vi "AudioTest.Run SoundCheck Sequence.vi"(7 "Config":T1={"SeqDir"=path "C:/MTE/Audio Test/Config/SoundCheck/Sequences", "SoundCheckApp"=path "C:/SoundCheck 16.0-x64/SoundCheck 16.0 (x64).exe", "IP"="localhost", "Port"=4444, "Process Name"="SoundCheck 16.0 (x64)", "DataDir"=path "C:/MTE/Audio Test/Data/SoundCheck", "Window"=enum."Normal"}, 8 "error in":errorcluster, 9 "UUT Dir":path, 10 "Timeout(s)":dbl=60.0, 11 "Sequence":string="UTAH_EV2_SEQUENCE_20180820_DUMMY2.sqc") -> (0 "error out":errorcluster, 1 "App Launch Dur(s)":dbl, 2 "Duration":dbl, 3 "Ran to completion":bool)   [LabVIEW 2018]
uses:
  TypeDefs/SoundCheck Config.ctl
  Common/Utils/Errors/Error.Error Code List.ctl
  <vilib>/KATE/Files/File Utils.lvlib
  <vilib>/KATE/Time/Time Utils.lvlib
panel:
  out "Status":string
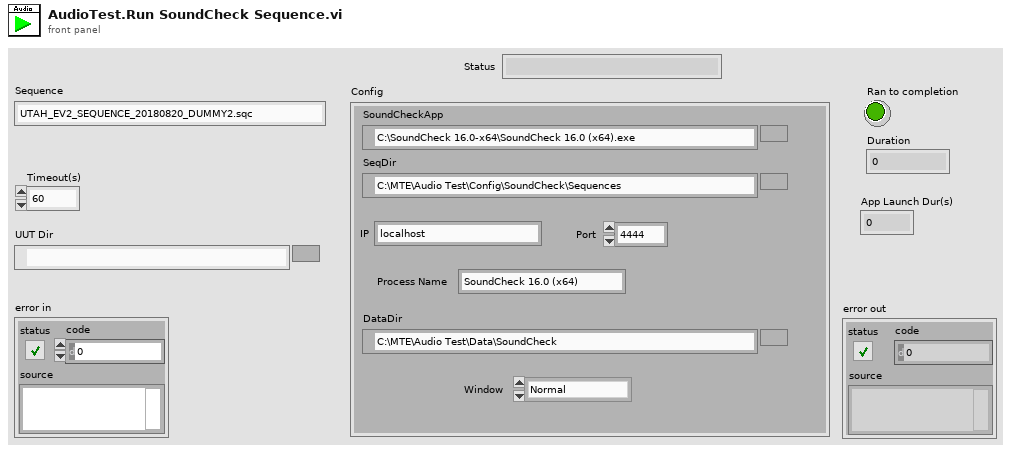
[diagram p1: front panel]
types:
  T1 = typedef "SoundCheck Config.ctl" = cluster{"SeqDir":path, "SoundCheckApp":path, "IP":string, "Port":u16, "Process Name":string, "DataDir":path, "Window":enum16{"Normal", "Minimized", "Hidden"}}
  T2 = typedef "Error.Error Code List.ctl" = i32
  T3 = cluster{"Config":T1, "Sequence":string, "Timeout(s)":dbl, "UUT Dir":path}
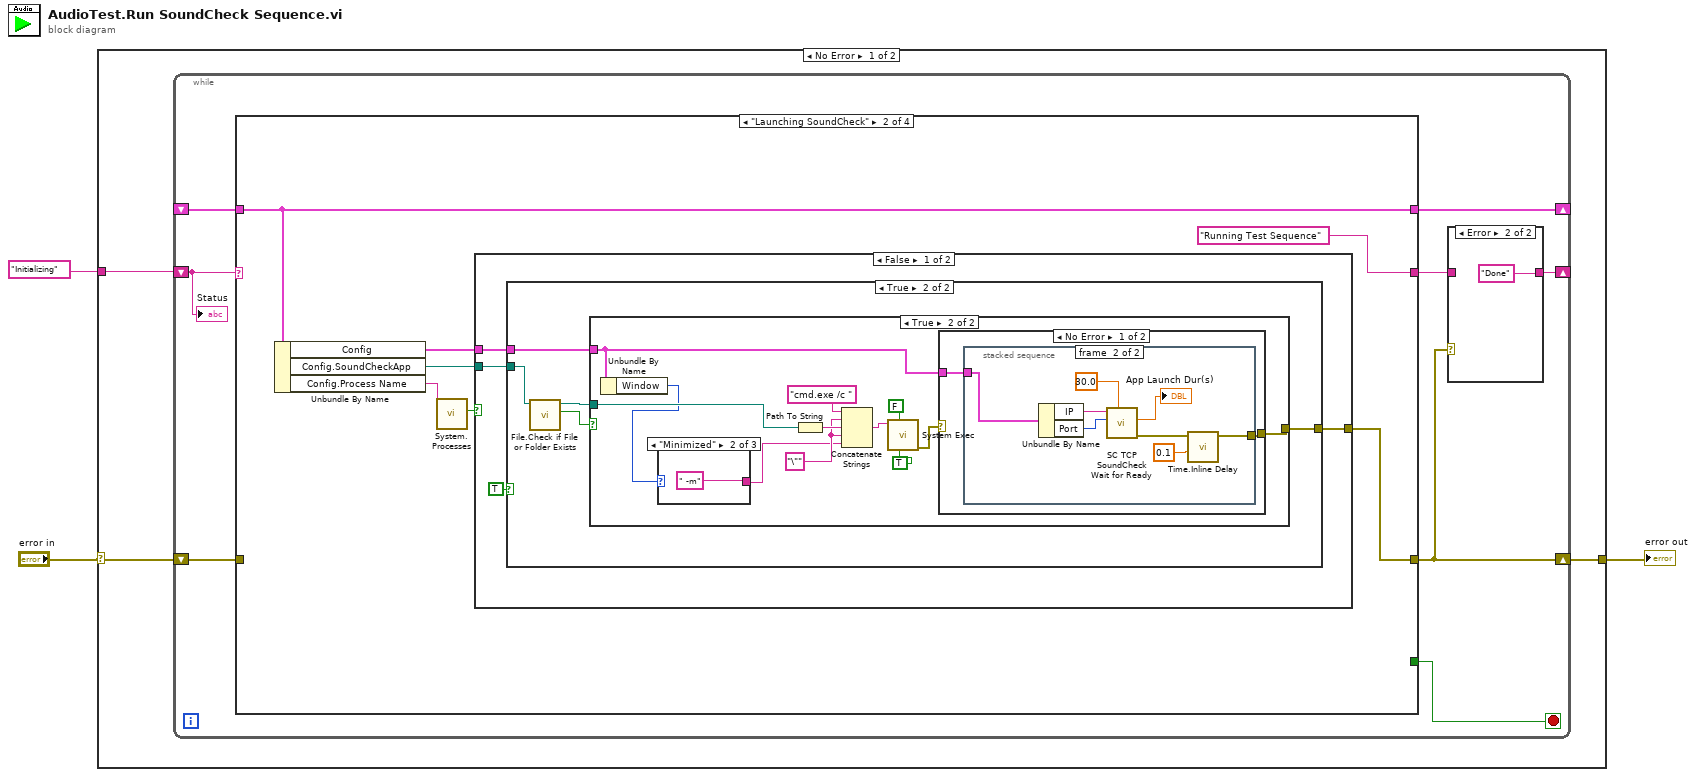
[diagram p0: block diagram]
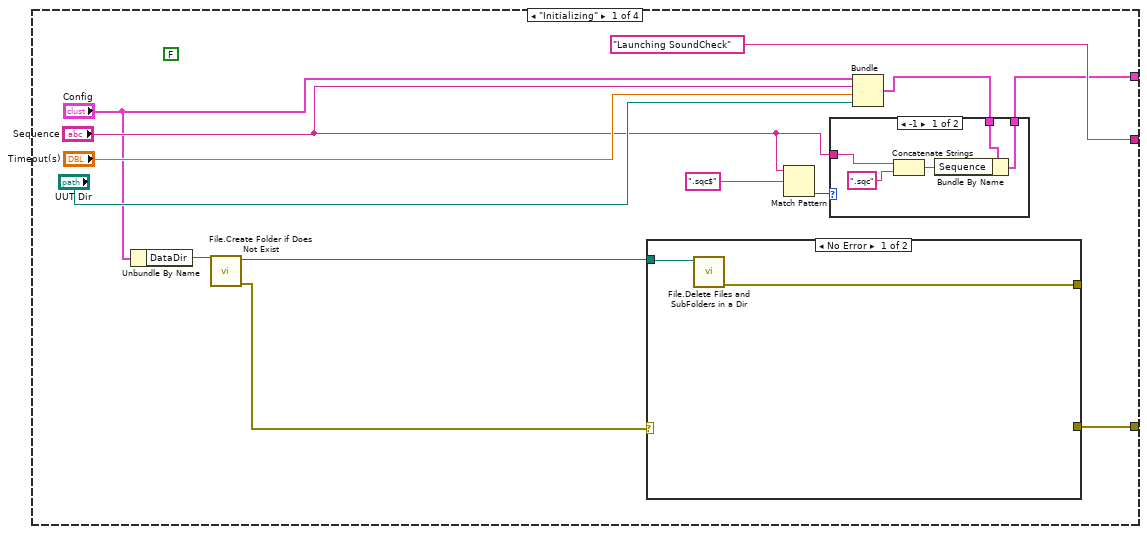
[diagram p3: hidden frame]
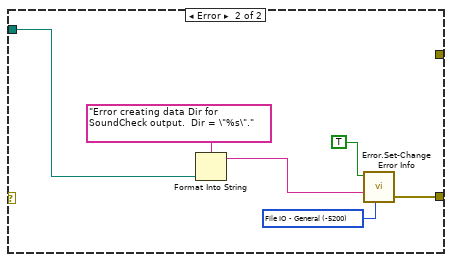
[diagram p5: hidden frame]
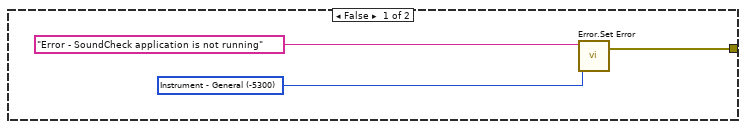
[diagram p6: hidden frame]
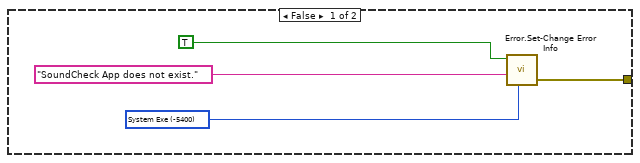
[diagram p7: hidden frame]
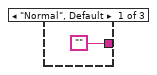
[diagram p8: hidden frame]
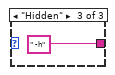
[diagram p9: hidden frame]
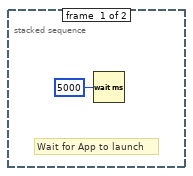
[diagram p10: hidden frame]
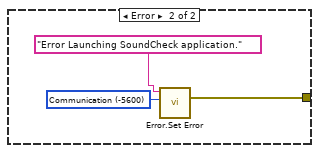
[diagram p11: hidden frame]
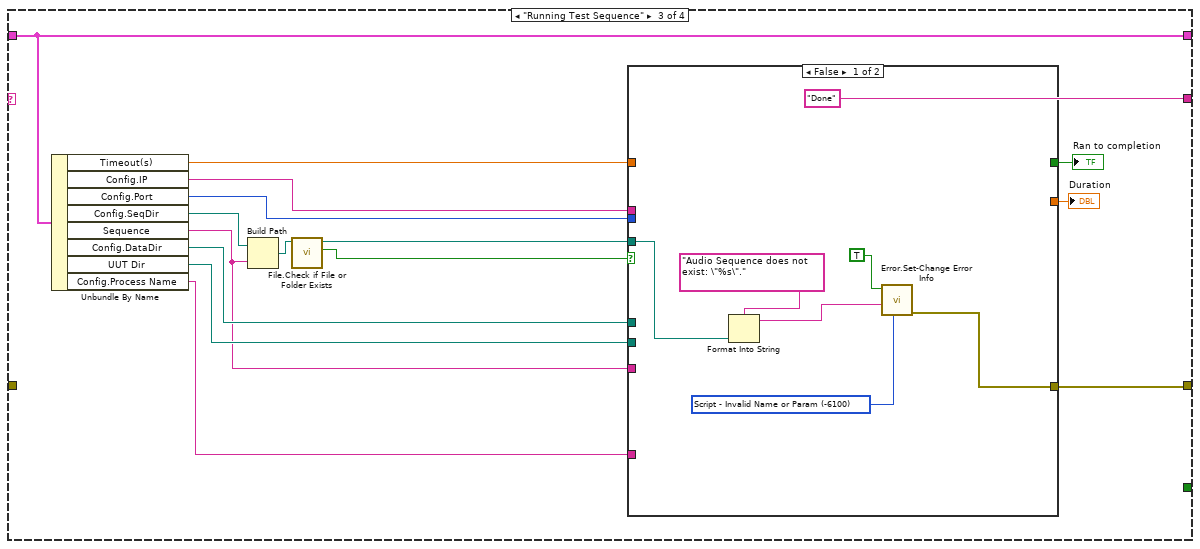
[diagram p13: hidden frame]
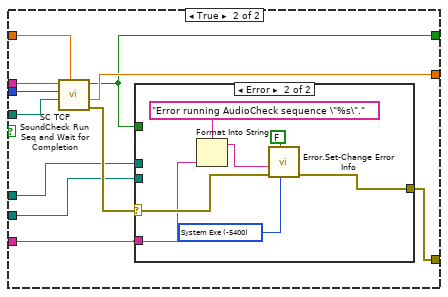
[diagram p14: hidden frame]
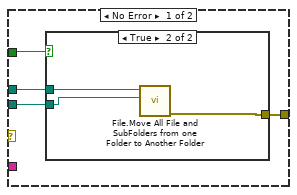
[diagram p15: hidden frame]
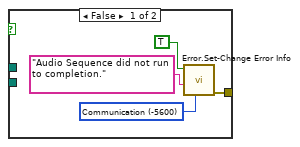
[diagram p16: hidden frame]
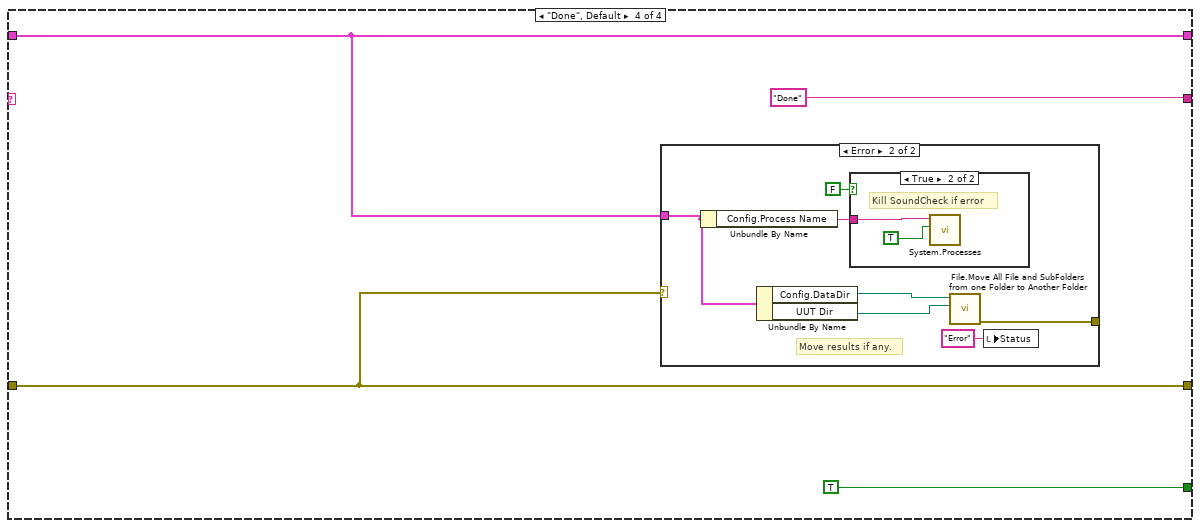
[diagram p17: hidden frame]
diagram:
  n1 = case shown="No Error" "error in" {
    selector: "error in" -> [w5 w160]
    tunnel: [w6 w160] -> w3
    tunnel: "Initializing" -> [w4 _]
    frame No Error {
      n2 = while {
        shift-right: [w14] -> _
        shift-left: _ -> [w13]
        shift-right: [w10] -> w6
        shift-left: w5 -> [w12]
        shift-right: [w8] -> _
        shift-left: w4 -> [w7]
        stop <- w11 stop-if-true
        n3 = case shown="\"Launching SoundCheck\"" w7 {
          tunnel: [w19 w48 w110 w148] -> w14
          tunnel: w13 -> [_ w48 w110 w148]
          tunnel: ["Launching SoundCheck" "Running Test Sequence" "Done" "Done"] -> w9
          tunnel: w12 -> [_ _ _ w147]
          tunnel: [w24 w49 w102 w147] -> w10
          tunnel: [_ _ _ TRUE] -> w11
          frame "Initializing" {
            (unwired) FALSE ("Done")
            n4 = Unbundle By Name("Config") -> ("DataDir"=w26:path)
            n5 = call <vilib>:"File.Create Folder if Does Not Exist.vi"("Path"=w26) -> ("error out"=w25:errorcluster, "Dup Path"=w18:path)  [unwired: 8 in, 1 out]
            n6 = case shown="No Error" w25 {
              tunnel: [_ w41] -> w24
              tunnel: w18 -> [w37 w39]
              tunnel: [w36 _] -> _
              frame No Error {
                n7 = call <vilib>:"File.Delete Files and SubFolders in a Dir.vi"("Dir"=w37) -> ("error out"=w36:errorcluster)  [unwired: 9 in, 1 out]
              }
              frame Error {
                w43 = T2 -5200 items=["No Error"=0, "Abort"=-2, "Misc"=-5000, "Fixture Error"=-5100, "File IO - General"=-5200, "FIle IO - Config Error"=-5201, "Instrument - General"=-5300, "Instrument - Serial Com"=-5301, "Instrument - Camera"=-5302, "Instrument - PS"=-5303, "Instrument - Oscilloscope"=-5304, "Instrument - Function Gen"=-5305, "Instrument - Load"=-5306, "Instrument - Meter"=-5307, "Instrument - Power Control"=-5308, "Instrument - Motion"=-5309, "Instrument - RF"=-5310, "System Exe"=-5400, "Image Processing"=-5500, "Communication"=-5600, "Script - Syntax Error"=-6000, "Script - Invalid Name or Param"=-6100, "Script - Timeout"=-6200, "Invalid Data"=-6300, "FW Update Error"=-6500] ("Std Code")
                n8 = Format Into String(format string="Error creating data Dir for SoundCheck output.  Dir = \"%s\"." ("Description"), w39) -> (resulting string=w38:string)  [unwired: 2 in, 1 out]
                n9 = call "Error.Set-Change Error Info.vi"("Std Code"=w43, "Description"=w38, "Set Error"=TRUE) -> ("error out"=w41:errorcluster)  [unwired: 8 in]
              }
            }
            n10 = Match Pattern(string="Sequence", regular expression=".sqc$") -> (offset past match=w22:i32)  [unwired: 1 in, 3 out]
            n11 = Bundle("Config"="Config", "Sequence"="Sequence", "Timeout(s)"="Timeout(s)", "UUT Dir"="UUT Dir") -> (w20:T3)  [unwired: 1 in]
            n12 = case shown="-1" w22 {
              tunnel: "Sequence" -> [w31 _]
              tunnel: w20 -> [w34 w35]
              tunnel: [w33 w35] -> w19
              frame -1 {
                n13 = Concatenate Strings(w31, ".sqc") -> (w32:string)
                n14 = Bundle By Name(cluster=w34, "Sequence"=w32) -> (w33:T3)
              }
              frame 0, Default {
              }
            }
          }
          frame "Launching SoundCheck" {
            n15 = Unbundle By Name(w48) -> ("Config"=w44:T1, "Config.SoundCheckApp"=w46:path, "Config.Process Name"=w47:string)
            n16 = call "System.Processes.vi"("Process Name"=w47) -> ("Is Running"=w45:bool)  [unwired: 8 in, 2 out]
            n17 = case shown="False" w45 {
              tunnel: [w54 _] -> w49
              tunnel: w46 -> [w53 _]
              tunnel: w44 -> [w52 _]
              frame False {
                n18 = case shown="True" TRUE {
                  tunnel: [w55 w62] -> w54
                  tunnel: w53 -> [_ w61]
                  tunnel: w52 -> [_ w58]
                  frame False {
                    w56 = T2 -5300 items=["No Error"=0, "Abort"=-2, "Misc"=-5000, "Fixture Error"=-5100, "File IO - General"=-5200, "FIle IO - Config Error"=-5201, "Instrument - General"=-5300, "Instrument - Serial Com"=-5301, "Instrument - Camera"=-5302, "Instrument - PS"=-5303, "Instrument - Oscilloscope"=-5304, "Instrument - Function Gen"=-5305, "Instrument - Load"=-5306, "Instrument - Meter"=-5307, "Instrument - Power Control"=-5308, "Instrument - Motion"=-5309, "Instrument - RF"=-5310, "System Exe"=-5400, "Image Processing"=-5500, "Communication"=-5600, "Script - Syntax Error"=-6000, "Script - Invalid Name or Param"=-6100, "Script - Timeout"=-6200, "Invalid Data"=-6300, "FW Update Error"=-6500] ("Std Code")
                    n19 = call "Error.Set Error.vi"("Code"=w56, "Desc"="Error - SoundCheck application is not running") -> ("error out"=w55:errorcluster)  [unwired: 5 in]
                  }
                  frame True {
                    n20 = call <vilib>:"File.Check if File or Folder Exists.vi"("Path"=w61) -> ("Exists"=w59:bool, "Dup Path"=w60:path)  [unwired: 6 in, 3 out]
                    n21 = case shown="True" w59 {
                      tunnel: [w66 w78] -> w62
                      tunnel: w60 -> [_ w70]
                      tunnel: w58 -> [_ w77]
                      frame False {
                        w63 = T2 -5400 items=["No Error"=0, "Abort"=-2, "Misc"=-5000, "Fixture Error"=-5100, "File IO - General"=-5200, "FIle IO - Config Error"=-5201, "Instrument - General"=-5300, "Instrument - Serial Com"=-5301, "Instrument - Camera"=-5302, "Instrument - PS"=-5303, "Instrument - Oscilloscope"=-5304, "Instrument - Function Gen"=-5305, "Instrument - Load"=-5306, "Instrument - Meter"=-5307, "Instrument - Power Control"=-5308, "Instrument - Motion"=-5309, "Instrument - RF"=-5310, "System Exe"=-5400, "Image Processing"=-5500, "Communication"=-5600, "Script - Syntax Error"=-6000, "Script - Invalid Name or Param"=-6100, "Script - Timeout"=-6200, "Invalid Data"=-6300, "FW Update Error"=-6500] ("Std Code")
                        n22 = call "Error.Set-Change Error Info.vi"("Std Code"=w63, "Description"="SoundCheck App does not exist.", "Set Error"=TRUE) -> ("error out"=w66:errorcluster)  [unwired: 8 in]
                      }
                      frame True {
                        w71 = "\"" ("string")
                        n23 = Unbundle By Name(w77) -> ("Window"=w68:enum16{"Normal", "Minimized", "Hidden"})
                        n24 = case shown="\"Minimized\"" w68 {
                          tunnel: ["" " -m" " -h"] -> w69
                          frame "Normal", Default {
                          }
                          frame "Minimized" {
                          }
                          frame "Hidden" {
                          }
                        }
                        n25 = Path To String(path=w70) -> (string=w72:string)
                        n26 = Concatenate Strings("cmd.exe /c ", w71, w72, w71, w69) -> (w76:string)
                        n27 = call <vilib>:"System Exec.vi"("run minimized? (F)"=TRUE, "wait until completion? (T)"=FALSE, "command line"=w76) -> ("error out"=w67:errorcluster)  [unwired: 5 in, 3 out]
                        n28 = case shown="No Error" w67 {
                          tunnel: [w82 w93] -> w78
                          tunnel: w77 -> [w83 _]
                          frame No Error {
                            n29 = stacked-sequence {
                              tunnel: w83 -> [_ w92]
                              tunnel: [_ w87] -> w82
                              frame #0 {
                                # "Wait for App to launch"
                                n30 = Wait (ms)(milliseconds to wait=u32 5000) -> ()  [unwired: 1 out]
                              }
                              frame #1 {
                                n31 = Unbundle By Name(w92) -> ("IP"=w91:string, "Port"=w90:u16)
                                n32 = call "SC TCP SoundCheck Wait for Ready.vi"("TimeOut(s)"=30.0, "port (4444)"=w90, "SoundCheck IP Address (localhost)"=w91) -> ("error out"=w88:errorcluster, "Duration"=→"App Launch Dur(s)":dbl)  [unwired: 6 in, 1 out]
                                n33 = call <vilib>:"Time.Inline Delay.vi"("Wait(secs)"=0.1, "error in top"=w88) -> ("error out top"=w87:errorcluster)  [unwired: 8 in, 1 out]
                              }
                            }
                          }
                          frame Error {
                            w95 = T2 -5600 items=["No Error"=0, "Abort"=-2, "Misc"=-5000, "Fixture Error"=-5100, "File IO - General"=-5200, "FIle IO - Config Error"=-5201, "Instrument - General"=-5300, "Instrument - Serial Com"=-5301, "Instrument - Camera"=-5302, "Instrument - PS"=-5303, "Instrument - Oscilloscope"=-5304, "Instrument - Function Gen"=-5305, "Instrument - Load"=-5306, "Instrument - Meter"=-5307, "Instrument - Power Control"=-5308, "Instrument - Motion"=-5309, "Instrument - RF"=-5310, "System Exe"=-5400, "Image Processing"=-5500, "Communication"=-5600, "Script - Syntax Error"=-6000, "Script - Invalid Name or Param"=-6100, "Script - Timeout"=-6200, "Invalid Data"=-6300, "FW Update Error"=-6500] ("Std Code")
                            n34 = call "Error.Set Error.vi"("Code"=w95, "Desc"="Error Launching SoundCheck application.") -> ("error out"=w93:errorcluster)  [unwired: 5 in]
                          }
                        }
                      }
                    }
                  }
                }
              }
              frame True {
                # "Do nothing\nAlready running"
              }
            }
          }
          frame "Running Test Sequence" {
            n35 = Unbundle By Name(w110) -> ("Timeout(s)"=w108:dbl, "Config.IP"=w109:string, "Config.Port"=w107:u16, "Config.SeqDir"=w106:path, "Sequence"=w96:string, "Config.DataDir"=w100:path, "UUT Dir"=w99:path, "Config.Process Name"=w97:string)
            n36 = Build Path(base path=w106, name or relative path=w96) -> (appended path=w105:path)
            n37 = call <vilib>:"File.Check if File or Folder Exists.vi"("Path"=w105) -> ("Exists"=w98:bool, "Dup Path"=w104:path)  [unwired: 6 in, 3 out]
            n38 = case shown="False" w98 {
              tunnel: w109 -> [_ w128]
              tunnel: w108 -> [_ w127]
              tunnel: w107 -> [_ w126]
              tunnel: w104 -> [w114 w125]
              tunnel: [_ w124] -> w103
              tunnel: [w116 w122] -> w102
              tunnel: [_ w121] -> w101
              tunnel: w100 -> [_ w120]
              tunnel: w99 -> [_ w119]
              tunnel: w97 -> [_ _]
              tunnel: w96 -> [_ w118]
              frame False {
                w117 = T2 -6100 items=["No Error"=0, "Abort"=-2, "Misc"=-5000, "Fixture Error"=-5100, "File IO - General"=-5200, "FIle IO - Config Error"=-5201, "Instrument - General"=-5300, "Instrument - Serial Com"=-5301, "Instrument - Camera"=-5302, "Instrument - PS"=-5303, "Instrument - Oscilloscope"=-5304, "Instrument - Function Gen"=-5305, "Instrument - Load"=-5306, "Instrument - Meter"=-5307, "Instrument - Power Control"=-5308, "Instrument - Motion"=-5309, "Instrument - RF"=-5310, "System Exe"=-5400, "Image Processing"=-5500, "Communication"=-5600, "Script - Syntax Error"=-6000, "Script - Invalid Name or Param"=-6100, "Script - Timeout"=-6200, "Invalid Data"=-6300, "FW Update Error"=-6500] ("Std Code")
                n39 = Format Into String(format string="Audio Sequence does not exist: \"%s\"." ("Description"), w114) -> (resulting string=w113:string)  [unwired: 2 in, 1 out]
                n40 = call "Error.Set-Change Error Info.vi"("Std Code"=w117, "Description"=w113, "Set Error"=TRUE) -> ("error out"=w116:errorcluster)  [unwired: 8 in]
              }
              frame True {
                n41 = call "SC TCP SoundCheck Run Seq and Wait for Completion.vi"("TimeOut(s)"=w127, "Sequence to run (full path)"=w125, "port (4444)"=w126, "SoundCheck IP Address (localhost)"=w128) -> ("error out"=w123:errorcluster, "Duration"=w124:dbl, "Ran to completion"=w121:bool)  [unwired: 5 in]
                n42 = case shown="Error" w123 {
                  selector: w123 -> [_ w146]
                  tunnel: [w131 w144] -> w122
                  tunnel: w121 -> [w132 _]
                  tunnel: w120 -> [w130 _]
                  tunnel: w119 -> [w129 _]
                  tunnel: w118 -> [_ w141]
                  frame No Error {
                    n43 = case shown="True" w132 {
                      tunnel: [w133 w137] -> w131
                      tunnel: w130 -> [_ w139]
                      tunnel: w129 -> [_ w138]
                      frame False {
                        w136 = T2 -5600 items=["No Error"=0, "Abort"=-2, "Misc"=-5000, "Fixture Error"=-5100, "File IO - General"=-5200, "FIle IO - Config Error"=-5201, "Instrument - General"=-5300, "Instrument - Serial Com"=-5301, "Instrument - Camera"=-5302, "Instrument - PS"=-5303, "Instrument - Oscilloscope"=-5304, "Instrument - Function Gen"=-5305, "Instrument - Load"=-5306, "Instrument - Meter"=-5307, "Instrument - Power Control"=-5308, "Instrument - Motion"=-5309, "Instrument - RF"=-5310, "System Exe"=-5400, "Image Processing"=-5500, "Communication"=-5600, "Script - Syntax Error"=-6000, "Script - Invalid Name or Param"=-6100, "Script - Timeout"=-6200, "Invalid Data"=-6300, "FW Update Error"=-6500] ("Std Code")
                        n44 = call "Error.Set-Change Error Info.vi"("Std Code"=w136, "Description"="Audio Sequence did not run to completion.", "Set Error"=TRUE) -> ("error out"=w133:errorcluster)  [unwired: 8 in]
                      }
                      frame True {
                        n45 = call "File.Move All File and SubFolders from one Folder to Another Folder.vi"("Destination Folder"=w138, "Source Folder"=w139) -> ("error out"=w137:errorcluster)  [unwired: 8 in, 1 out]
                      }
                    }
                  }
                  frame Error {
                    w145 = T2 -5400 items=["No Error"=0, "Abort"=-2, "Misc"=-5000, "Fixture Error"=-5100, "File IO - General"=-5200, "FIle IO - Config Error"=-5201, "Instrument - General"=-5300, "Instrument - Serial Com"=-5301, "Instrument - Camera"=-5302, "Instrument - PS"=-5303, "Instrument - Oscilloscope"=-5304, "Instrument - Function Gen"=-5305, "Instrument - Load"=-5306, "Instrument - Meter"=-5307, "Instrument - Power Control"=-5308, "Instrument - Motion"=-5309, "Instrument - RF"=-5310, "System Exe"=-5400, "Image Processing"=-5500, "Communication"=-5600, "Script - Syntax Error"=-6000, "Script - Invalid Name or Param"=-6100, "Script - Timeout"=-6200, "Invalid Data"=-6300, "FW Update Error"=-6500] ("Std Code")
                    n46 = Format Into String(format string="Error running AudioCheck sequence \"%s\"." ("Description"), w141) -> (resulting string=w142:string)  [unwired: 2 in, 1 out]
                    n47 = call "Error.Set-Change Error Info.vi"("Std Code"=w145, "Append Details"=FALSE, "error in"=w146, "Description"=w142) -> ("error out"=w144:errorcluster)  [unwired: 7 in]
                  }
                }
              }
            }
            "Duration" <- w103
            "Ran to completion" <- w101
          }
          frame "Done", Default {
            n48 = case shown="Error" w147 {
              tunnel: w148 -> [_ w153]
              tunnel: [_ w152] -> _
              frame No Error {
              }
              frame Error {
                # "Move results if any."
                n49 = Unbundle By Name(w153) -> ("Config.Process Name"=w157:string)
                n50 = Unbundle By Name(w153) -> ("Config.DataDir"=w154:path, "UUT Dir"=w155:path)
                n51 = case shown="True" FALSE {
                  tunnel: w157 -> [_ w159]
                  frame False {
                  }
                  frame True {
                    # "Kill SoundCheck if error"
                    n52 = call "System.Processes.vi"("Kill"=TRUE, "Process Name"=w159) -> ()  [unwired: 7 in, 3 out]
                  }
                }
                n53 = call "File.Move All File and SubFolders from one Folder to Another Folder.vi"("Destination Folder"=w155, "Source Folder"=w154) -> ("error out"=w152:errorcluster)  [unwired: 8 in, 1 out]
                n54 = local write "Status"("Error" ("Status")) -> ()
              }
            }
          }
        }
        n55 = case shown="Error" w10 {
          tunnel: w9 -> [w15 _]
          tunnel: [w15 "Done"] -> w8
          frame No Error {
          }
          frame Error {
          }
        }
        "Status" <- w7
      }
    }
    frame Error {
    }
  }
  "error out" <- w3
